vi "processSysSubscription.vi"(8 "error in (no error)":errorcluster, 9 "Message":string, 10 "Topic":string, 11 "MQTTclient in":refnum<class "MQTTclient.lvclass">) -> (0 "error out":errorcluster, 1 "Message":string, 2 "Topic":string, 3 "MQTTclient out":refnum<class "MQTTclient.lvclass">, 5 "Send?":bool)   [LabVIEW 2017, in "MQTTclient.lvclass"]
uses:
  MQTTclient.lvclass
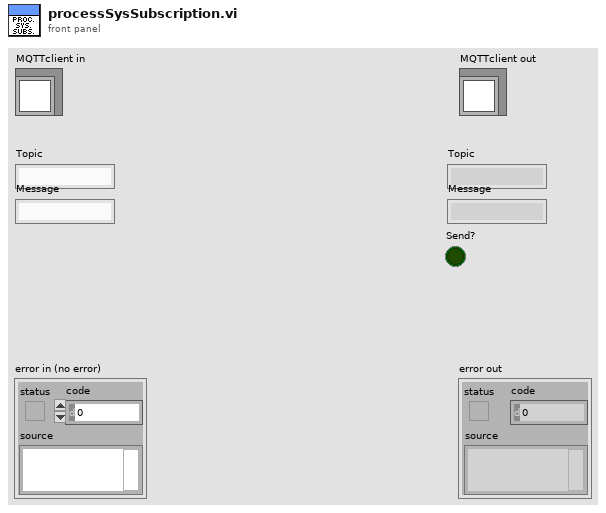
[diagram p1: front panel]
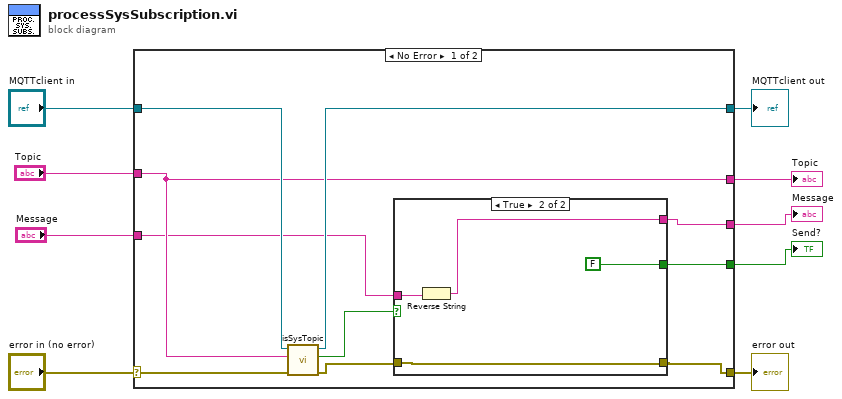
[diagram p0: block diagram]
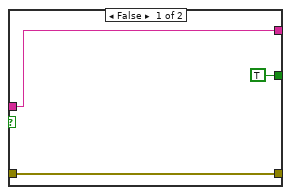
[diagram p2: hidden frame]
diagram:
  n1 = case shown="No Error" "error in (no error)" {
    selector: "error in (no error)" -> [w19 w28]
    tunnel: [w13 w28] -> w8
    tunnel: [w17 w27] -> w6
    tunnel: "MQTTclient in" -> [w18 w27]
    tunnel: "Topic" -> [w16 _]
    tunnel: [w16 _] -> w4
    tunnel: [w11 _] -> w3
    tunnel: "Message" -> [w14 _]
    tunnel: [w10 _] -> w1
    frame No Error {
      n2 = call-dynamic "isSysTopic.vi"("error in (no error)"=w19, "Topic"=w16, "MQTTclient in"=w18) -> ("error out"=w12:errorcluster, "isSys?"=w15:bool, "MQTTclient out"=w17:refnum<class "MQTTclient.lvclass">)  [unwired: 6 in]
      n3 = case shown="True" w15 {
        tunnel: w14 -> [w22 w25]
        tunnel: [w20 w26] -> w13
        tunnel: w12 -> [w20 w26]
        tunnel: [w22 w24] -> w11
        tunnel: [TRUE ("Send?") FALSE ("Send?")] -> w10
        frame False {
        }
        frame True {
          n4 = Reverse String(1:w25) -> (0:w24:string)
        }
      }
    }
    frame Error {
    }
  }
  "error out" <- w8
  "MQTTclient out" <- w6
  "Topic" <- w4
  "Message" <- w3
  "Send?" <- w1
